vi "xiC - PLAY.vi"(6 "Data":variant, 8 "error in (no error)":errorcluster, 11 "Attributes In":T1) -> (0 "error out":errorcluster, 3 "Attributes In":T1)   [LabVIEW 2013]
uses:
  xiC - Attributes.ctl
  C:/Projects/Cameras3.x/xiLib/xiLIB_64bit/xiLIB/xiCamLib/API/x64/xiApi.NETX64.dll
  xiLIB_64bit/xiLIB/xiCamLib/API/x64/xiApi.NETX64.dll
  xiC - TreeDisplayType.ctl
  <vilib>/Utility/High Resolution Relative Seconds.vi
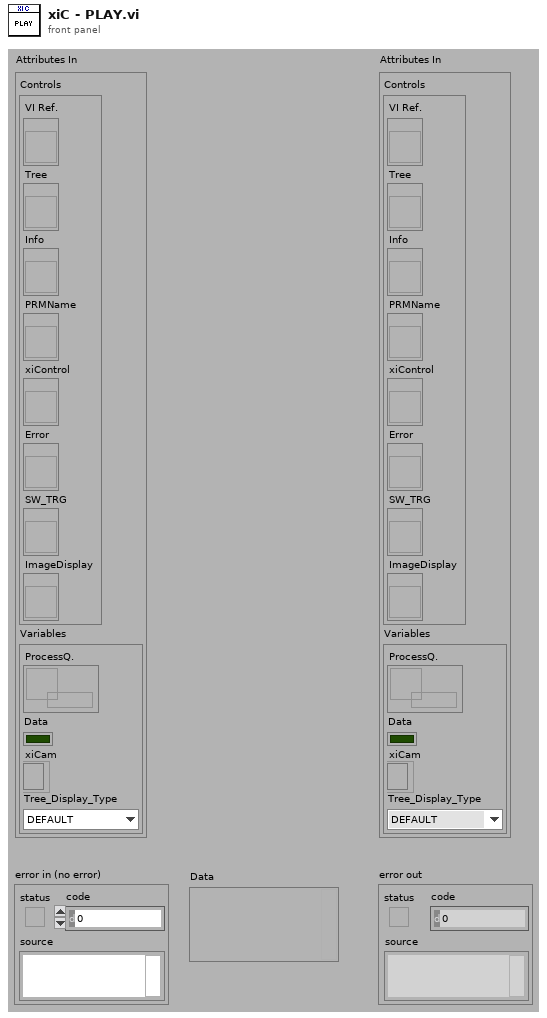
[diagram p1: front panel]
types:
  T1 = typedef "xiC - Attributes.ctl" = cluster{"Controls":cluster{"VI Ref.":refnum<vi>, "Tree":refnum<vi>, "Info":refnum<vi>, "PRMName":refnum<vi>, "xiControl":refnum<vi>, "Error":refnum<vi>, "SW_TRG":refnum<vi>, "ImageDisplay":refnum<vi>}, "Variables":cluster{"ProcessQ.":refnum<queue>, "Data":bool, "xiCam":refnum<k24>, "Tree_Display_Type":T2}}
  T2 = typedef "xiC - TreeDisplayType.ctl" = enum16{"DEFAULT", "HIDE_MAX_MIN"}
  T3 = typedef "xiImageMng - Attributes.ctl" = cluster{"WIDTH":i32, "HEIGHT":i32, "IMG_FORMAT":T4}
  T4 = typedef "IMG_DATA_FORMAT.ctl" = enum16{"MONO8", "MONO16", "RGB24", "RGB32", "RGBPLANAR", "RAW8", "RAW16"}
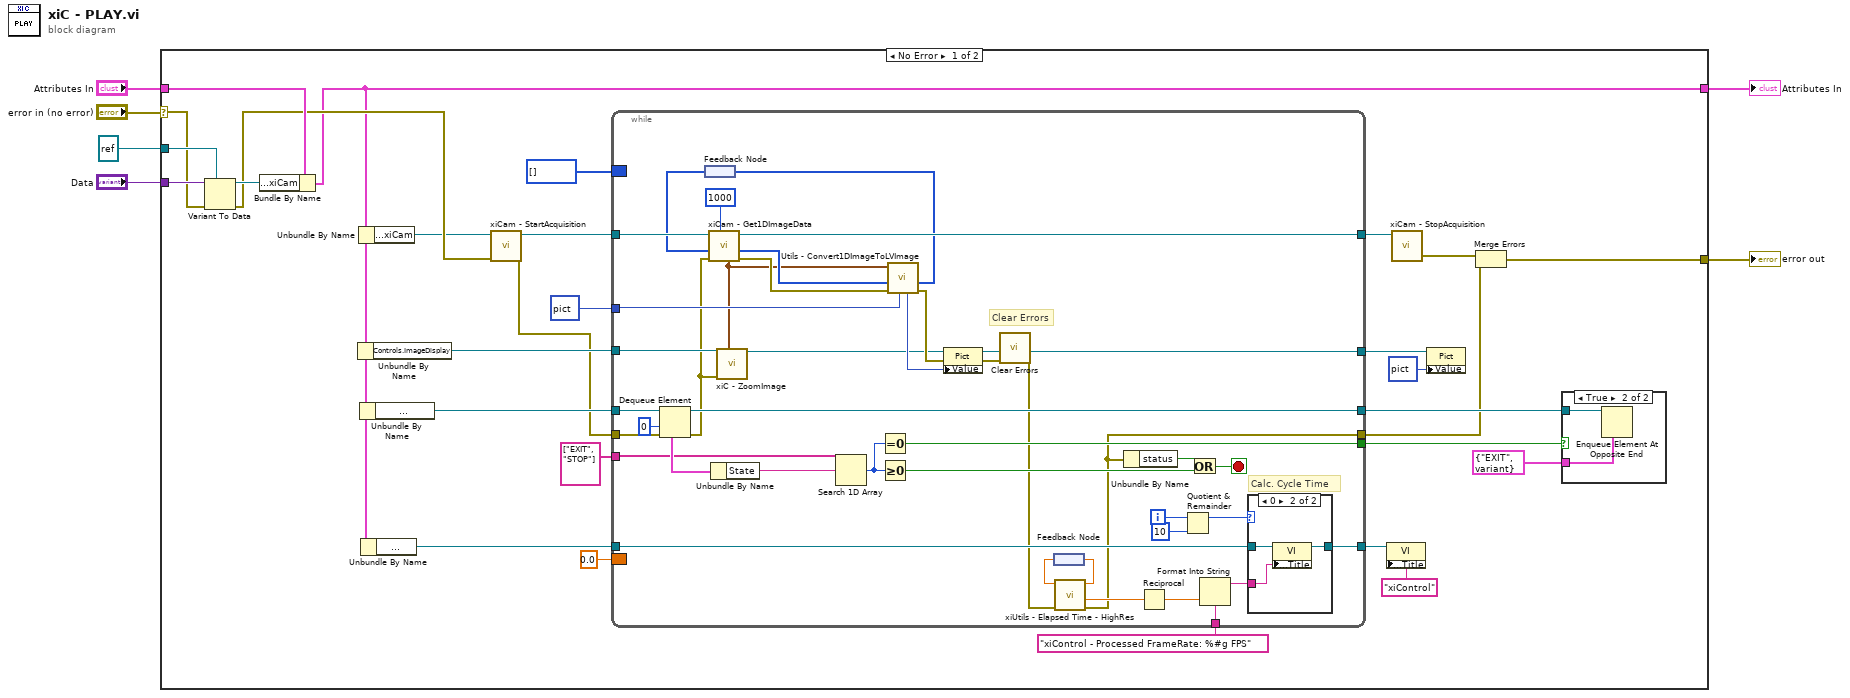
[diagram p0: block diagram]
diagram:
  n1 = case shown="No Error" "error in (no error)" {
    selector: "error in (no error)" -> [w14 w84]
    tunnel: [w22 w84] -> w6
    tunnel: "Attributes In" -> [w15 w83]
    tunnel: [w12 w83] -> w4
    tunnel: "Data" -> [w18 _]
    tunnel: refnum<k24> refnum ("Variables.xiCam") -> [w17 _]
    frame No Error {
      n2 = Variant To Data(error in=w14, type=w17, Variant=w18) -> (data=w16:refnum<k24>, error out=w13:errorcluster)
      n3 = Bundle By Name(cluster=w15, "Variables.xiCam"=w16) -> (w12:T1)
      n4 = Unbundle By Name(w12) -> ("Controls.ImageDisplay"=w26:refnum<vi>)
      n5 = Unbundle By Name(w12) -> ("Variables.xiCam"=w11:refnum<k24>)
      n6 = Unbundle By Name(w12) -> ("Variables.ProcessQ."=w35:refnum<queue>)
      n7 = Unbundle By Name(w12) -> ("Controls.VI Ref."=w29:refnum<vi>)
      n8 = call "xiCam - StartAcquisition.vi"("error in (no error)"=w13, "xiCam In"=w11) -> ("error out"=w9:errorcluster, "xiCam Out"=w27:refnum<k24>)  [unwired: 8 in]
      n9 = while {
        tunnel: w35 -> [w78]
        tunnel: w9 -> [w77]
        tunnel: string[] ["EXIT", "STOP"] -> [w73]
        tunnel: [w50] -> w23
        tunnel: [w69] -> w33
        tunnel: [w68] -> w32
        border: 0.0 ("Tick (ms) In") -> [_]
        tunnel: w29 -> [w59]
        tunnel: "xiControl - Processed FrameRate: %#g FPS" ("format string") -> [w61]
        border: u8[] [] -> [_]
        tunnel: w27 -> [w57]
        tunnel: [w55] -> w25
        tunnel: w26 -> [w54]
        tunnel: [w53] -> w21
        tunnel: [w52] -> w20
        tunnel: picture data[5B] ("picture") -> [w41]
        i -> [w64]
        stop <- w71 stop-if-true
        # "Clear Errors"
        # "Calc. Cycle Time"
        n10 = Dequeue Element(queue=w78, timeout in ms (-1)=0, error in (no error)=w77) -> (queue out=w68:refnum<queue>, element=w75:cluster{"State":string, "Data":variant}, error out=w38:errorcluster)  [unwired: 1 out]
        n11 = feedback #1() -> (w56:u8[])
        n12 = call "xiCam - Get1DImageData.vi"("timeout"=1000, "error in (no error)"=w38, "1DImageData In"=w56, "xiCam In"=w57) -> ("error out"=w49:errorcluster, "1DImageData Out"=w44:u8[], "xiCam Out"=w55:refnum<k24>, "Image Properites"=w39:T3)  [unwired: 4 in]
        n13 = Unbundle By Name(w75) -> ("State"=w74:string)
        n14 = call "xiC - ZoomImage.vi"("Image Properites"=w39, "error in (no error)"=w38, "Picture in"=w54) -> ("Picture out"=w40:refnum<vi>)  [unwired: 7 in, 1 out]
        n15 = Search 1D Array(1D array=w73, element=w74) -> (index of element=w70:i32)  [unwired: 1 in]
        n16 = Equal To 0?(x=w70) -> (x = 0?=w69:bool)
        n17 = Greater Or Equal To 0?(x=w70) -> (x >= 0?=w72:bool)
        n18 = call "Utils - Convert1DImageToLVImage.vi"("picture"=w41, "error in (no error)"=w49, "1DImageData In"=w44, "Image Properties In"=w39) -> ("error out"=w45:errorcluster, "1DImageData Out"=w48:u8[], "new picture"=w46:picture)  [unwired: 5 in]
        n19 = feedback-in #1(w48) -> ()
        n20 = property class="Pict"(reference=w40, error in=w45, "Value"=w46) -> (reference out=w53:refnum<vi>, error out=w43:errorcluster)
        n21 = call <vilib>:"Clear Errors.vi"("error in (no error)"=w43) -> ("error out"=w42:errorcluster)  [unwired: 6 in]
        n22 = feedback #2() -> (w66:dbl)
        n23 = call "xiUtils - Elapsed Time - HighRes.vi"("error in (no error)"=w42, "Tick (ms) In"=w66) -> ("error out"=w50:errorcluster, "Elapsed Time(ms)"=w62:dbl, "Tick (ms) Out"=w67:dbl)  [unwired: 7 in]
        n24 = feedback-in #2(w67) -> ()
        n25 = Unbundle By Name(w50) -> ("status"=w58:bool)
        n26 = Reciprocal(x=w62) -> (1/x=w47:dbl)
        n27 = Quotient & Remainder(x=w64, y=10) -> (x-y*floor(x/y)=w63:i32)  [unwired: 1 out]
        n28 = Or(x=w58, y=w72) -> (x .or. y?=w71:bool)
        n29 = Format Into String(format string=w61, w47) -> (resulting string=w60:string)  [unwired: 2 in, 1 out]
        n30 = case shown="0" w63 {
          tunnel: w60 -> [_ w81]
          tunnel: w59 -> [w79 w82]
          tunnel: [w79 w80] -> w52
          frame Default {
          }
          frame 0 {
            n31 = property class="VI"(reference=w82, "Front Panel.Title"=w81) -> (reference out=w80:refnum<vi>)  [unwired: 1 in, 1 out]
          }
        }
      }
      n32 = property class="VI"(reference=w20, "Front Panel.Title"="xiControl" ("format string")) -> ()  [unwired: 1 in, 2 out]
      n33 = call "xiCam - StopAcquisition.vi"("xiCam In"=w25) -> ("error out"=w24:errorcluster)  [unwired: 9 in, 1 out]
      n34 = property class="Pict"(reference=w21, "Value"=picture data[5B]) -> ()  [unwired: 1 in, 2 out]
      n35 = Merge Errors(w24, w23) -> (w22:errorcluster)
      n36 = case shown="True" w33 {
        tunnel: w32 -> [_ w37]
        tunnel: cluster{"State":string, "Data":variant} {"State"="EXIT", "Data"=variant} ("element") -> [_ w36]
        frame False {
        }
        frame True {
          n37 = Enqueue Element At Opposite End(queue=w37, element=w36) -> ()  [unwired: 2 in, 3 out]
        }
      }
    }
    frame Error {
    }
  }
  "error out" <- w6
  "Attributes In" <- w4
